vi "ziSweeper.vi"(0 "Handle In":T1 {"Handle" format="0x%08x"; "Conn" format="0x%08x"}, 1 "Output Channel (6)":u16=6 max=7, 2 "Signal Output (0)":u16 max=1, 3 "Signal Input UNUSED(0)":u16 max=1, 5 "Sweep Sequence":dbl[][](array[numeric]) format="%#_6p", 7 "Oscillator (0)":u16, 9 "Averaging":u16(ring)=1 caption="Averaging (1)" items=["1"=1, "2"=2, "4"=4, "16"=16, "32"=32, "64"=64, "128"=128], 11 "Error In":errorcluster, 12 "Input Demods (0)":u16[](array[numeric])=[0], 13 "Harmonic (1=fundamental)":i32=1 min=1 max=66000, 14 "Order (4)":i32(ring)=4 items=["6, 1st"=1, "12, 2nd"=2, "18, 3rd"=3, "24, 4th"=4, "30, 5th"=5, "36, 6th"=6, "42, 7th"=7, "48, 8th"=8]) -> (4 "Handle Out":T1 {"Handle" format="0x%08x"; "Conn" format="0x%08x"}, 6 "Output (F,X1,Y1,X2,Y2,...,Vo)":dbl[][](array[numeric]) format="%#_4p", 15 "Error Out":errorcluster)   [LabVIEW 2009, in "Zurich Instruments LabOne.lvlib"]
doc: "Perform a frequency sweep with the speciefied paramters. Use <B>ziSweepGenerator.vi</B> to generate the <B>Sweep Sequence</B>.\n\n<B>Output Channel</B> selects the channel in the output mixer that is used to generate the signal. This also determines the respective demodulator for generation of a sinusoidal.\n\nNote: <B>Signal Input</B> is only supported with the HF2LI when the Multifrequency option is installed."
uses:
  <instrlib>/Zurich Instruments LabOne/Zurich Instruments LabOne.lvlib
  <instrlib>/Zurich Instruments LabOne/Public/ziTypeHandle.ctl
  <instrlib>/Zurich Instruments LabOne/Public/Utility/ziTicksToS_single.vi
panel:
  out "Graph":cluster{dbl[], dbl[]}[](graph)
  in  "Abort":bool
  out "Remaining settle (s)":dbl caption="time to next value"
  out "Frequency":dbl caption="Frequency (Hz)" format="%_7p"
  out "Point":i32 caption="Point (#)"
  out "Progress":dbl(slide) scale=0.0..1.0
  out "Bandwidth_indic":dbl=100.0 caption="Bandwidth (Hz)" format="%_3p"
  # "Status"
  # "Progress (%)"
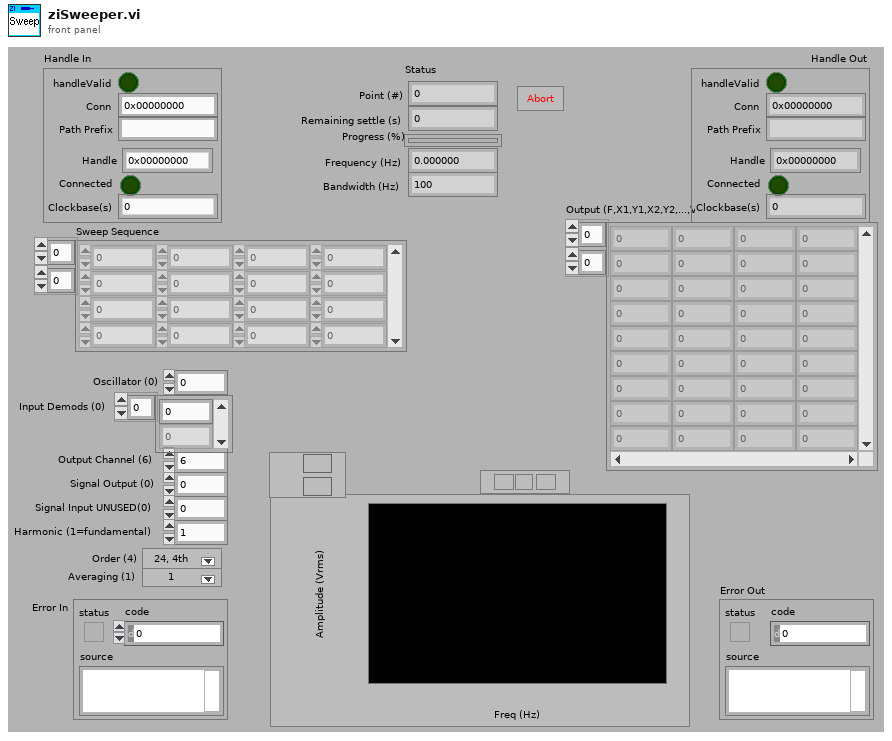
[diagram p1: front panel]
types:
  T1 = typedef "Zurich Instruments LabOne.lvlib/ziTypeHandle.ctl" = cluster{"handleValid":bool, "Conn":u64, "Path Prefix":string, "Handle":u64, "Connected":bool, "Clockbase(s)":dbl}
  T2 = cluster{"Timestamps (ticks)":u64, "X (Vrms)":dbl, "Y (Vrms)":dbl, "Osc Phase (deg)":dbl, "Freq (Hz)":dbl, "DIO":u32, "AuxIn0 (V)":dbl, "AuxIn1 (V)":dbl}
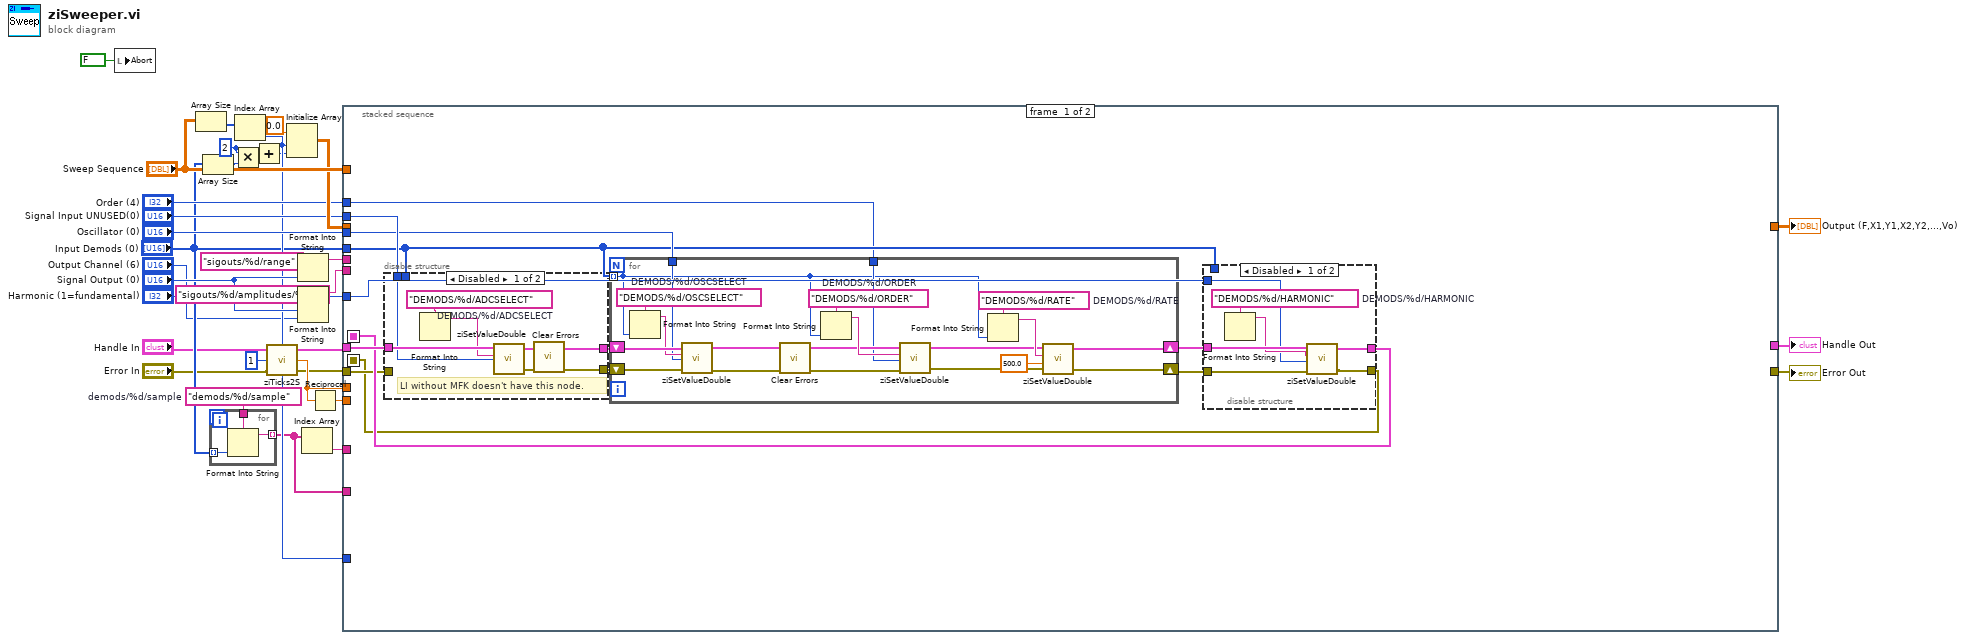
[diagram p0: block diagram]
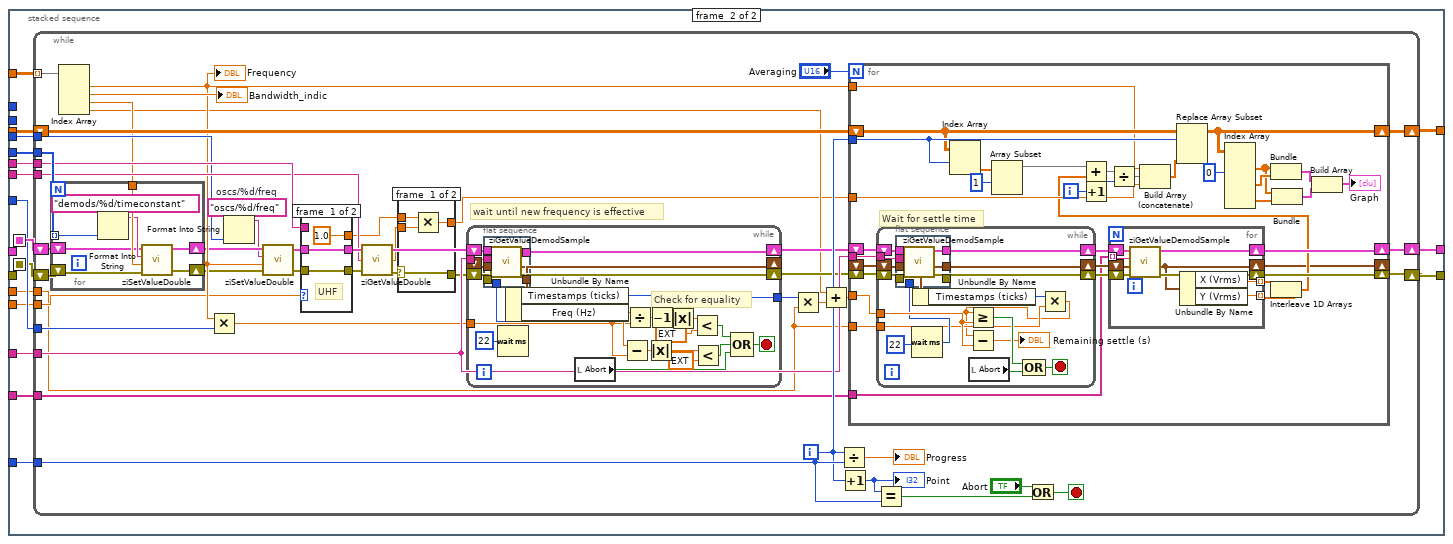
[diagram p4: hidden frame]
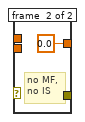
[diagram p5: hidden frame]
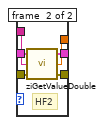
[diagram p6: hidden frame]
diagram:
  w16 = "demods/%d/sample"  # demods/%d/sample
  w9 = 2 ("dimension size")
  n1 = local write "Abort"(FALSE ("Abort")) -> ()
  n2 = Array Size(array="Sweep Sequence") -> (size(s)=w33:i32[])
  n3 = Array Size(array="Input Demods (0)") -> (size(s)=w11:i32)
  n4 = for {
    tunnel: w16 -> [w37]
    tunnel: "Input Demods (0)" -> [w36] mode=indexing
    tunnel: [w35] -> w14 mode=indexing
    n5 = Format Into String(format string=w37, w36) -> (resulting string=w35:string)  [unwired: 2 in, 1 out]
  }
  n6 = Multiply(x=w9, y=w11) -> (x*y=w10:i32)
  n7 = Index Array(array=w33) -> (element=w17:i32)  [unwired: 1 in]
  n8 = Add(x=w9, y=w10) -> (x+y=w13:i32)
  n9 = call-poly <instrlib>:"ziTicks2S.vi"("Error In"="Error In", "Timestamp(ticks)"=u64 1, "Handle In"="Handle In") -> ("Error Out"=w1:errorcluster, "Timestamp(s)"=w3:dbl, "Handle Out"=w5:T1)
  n10 = Initialize Array(0.0 ("dimension size"), w17, w13) -> (w31:dbl[][])
  n11 = Format Into String(format string="sigouts/%d/range", "Signal Output (0)") -> (resulting string=w29:string)  [unwired: 2 in, 1 out]
  n12 = Format Into String(format string="sigouts/%d/amplitudes/%d", "Signal Output (0)", "Output Channel (6)") -> (resulting string=w20:string)  [unwired: 2 in, 1 out]
  n13 = Index Array(array=w14) -> (element=w15:string)  [unwired: 1 in]
  n14 = Reciprocal(x=w3) -> (1/x=w7:dbl)
  n15 = stacked-sequence {
    seq-local: [w42 _] -> [_ w100]
    seq-local: [w39 _] -> [_ w90]
    tunnel: w31 -> [_ w104]
    tunnel: w5 -> [w50 _]
    tunnel: [_ w103] -> w25
    tunnel: [_ w102] -> w24
    tunnel: "Sweep Sequence" -> [_ w101]
    tunnel: "Input Demods (0)" -> [w46 w99]
    tunnel: w17 -> [_ w98]
    tunnel: w15 -> [_ w97]
    tunnel: w29 -> [_ w96]
    tunnel: w20 -> [_ w95]
    tunnel: [_ w94] -> w26
    tunnel: "Signal Input UNUSED(0)" -> [w48 _]
    tunnel: "Oscillator (0)" -> [w47 w92]
    tunnel: w1 -> [w40 _]
    tunnel: "Harmonic (1=fundamental)" -> [w38 w93]
    tunnel: "Order (4)" -> [w41 _]
    tunnel: w14 -> [_ w91]
    tunnel: w7 -> [_ w89]
    tunnel: w3 -> [_ w88]
    frame #0 {
      n16 = disable-structure shown="Disabled" {
        disable-tunnel: w50 -> [w56 w59]
        disable-tunnel: w48 -> [w54 _]
        disable-tunnel: w46 -> [_ _]
        disable-tunnel: [w52 w59] -> w44
        disable-tunnel: [w51 w58] -> w43
        disable-tunnel: w40 -> [_ w58]
        frame #0 {
          w57 = "DEMODS/%d/ADCSELECT"  # DEMODS/%d/ADCSELECT
          # "LI without MFK doesn't have this node."
          n17 = Format Into String(format string=w57) -> (resulting string=w55:string)  [unwired: 3 in, 1 out]
          n18 = call <instrlib>:"ziSetValueDouble.vi"("Value"=w54, "Path"=w55, "Handle In"=w56) -> ("Error Out"=w53:errorcluster, "Handle Out"=w52:T1)  [unwired: 2 in]
          n19 = call <vilib>:"Clear Errors.vi"("error in (no error)"=w53) -> ("error out"=w51:errorcluster)  [unwired: 6 in]
        }
        frame #1 {
        }
      }
      n20 = for {
        tunnel: w47 -> [w83]
        tunnel: w46 -> [w72] mode=indexing
        shift-right: [w71] -> w49
        shift-left: w44 -> [w86]
        shift-right: [w70] -> w45
        shift-left: w43 -> [w84]
        tunnel: w41 -> [w78]
        w75 = "DEMODS/%d/RATE"  # DEMODS/%d/RATE
        w82 = "DEMODS/%d/ORDER"  # DEMODS/%d/ORDER
        w87 = "DEMODS/%d/OSCSELECT"  # DEMODS/%d/OSCSELECT
        n21 = Format Into String(format string=w87, w72) -> (resulting string=w85:string)  [unwired: 2 in, 1 out]
        n22 = call <instrlib>:"ziSetValueDouble.vi"("Error In"=w84, "Value"=w83, "Path"=w85, "Handle In"=w86) -> ("Error Out"=w69:errorcluster, "Handle Out"=w80:T1)  [unwired: 1 in]
        n23 = call <vilib>:"Clear Errors.vi"("error in (no error)"=w69) -> ("error out"=w79:errorcluster)  [unwired: 6 in]
        n24 = Format Into String(format string=w82, w72) -> (resulting string=w81:string)  [unwired: 2 in, 1 out]
        n25 = call <instrlib>:"ziSetValueDouble.vi"("Error In"=w79, "Value"=w78, "Path"=w81, "Handle In"=w80) -> ("Error Out"=w74:errorcluster, "Handle Out"=w73:T1)  [unwired: 1 in]
        n26 = Format Into String(format string=w75, w72) -> (resulting string=w76:string)  [unwired: 2 in, 1 out]
        n27 = call <instrlib>:"ziSetValueDouble.vi"("Error In"=w74, "Value"=500.0 ("double precision float"), "Path"=w76, "Handle In"=w73) -> ("Error Out"=w70:errorcluster, "Handle Out"=w71:T1)  [unwired: 1 in]
      }
      n28 = disable-structure shown="Disabled" {
        disable-tunnel: w49 -> [w65 w68]
        disable-tunnel: w38 -> [w63 _]
        disable-tunnel: [w62 w68] -> w42
        disable-tunnel: [w61 w67] -> w39
        disable-tunnel: w46 -> [_ _]
        disable-tunnel: w45 -> [w60 w67]
        frame #0 {
          w66 = "DEMODS/%d/HARMONIC"  # DEMODS/%d/HARMONIC
          n29 = Format Into String(format string=w66) -> (resulting string=w64:string)  [unwired: 3 in, 1 out]
          n30 = call <instrlib>:"ziSetValueDouble.vi"("Error In"=w60, "Value"=w63, "Path"=w64, "Handle In"=w65) -> ("Error Out"=w61:errorcluster, "Handle Out"=w62:T1)  [unwired: 1 in]
        }
        frame #1 {
        }
      }
    }
    frame #1 {
      n31 = while {
        shift-right: [w152] -> w103
        shift-left: w100 -> [w115]
        shift-right: [w146] -> w102
        shift-left: w90 -> [w116]
        tunnel: w99 -> [w151]
        shift-right: [w148] -> w94
        shift-left: w104 -> [w134]
        tunnel: w101 -> [w147] mode=indexing
        tunnel: w98 -> [w137]
        tunnel: w97 -> [w130]
        tunnel: w96 -> [w145]
        tunnel: w95 -> [w144]
        tunnel: w93 -> [w143]
        tunnel: w92 -> [w142]
        tunnel: w91 -> [w114]
        tunnel: w89 -> [w106]
        tunnel: w88 -> [w105]
        i -> [w132]
        stop <- w138 stop-if-true
        w127 = "oscs/%d/freq"  # oscs/%d/freq
        # "wait until new frequency is effective"
        n32 = Index Array(array=w147) -> (element #1=w133:dbl, element #2=→"Bandwidth_indic":dbl, element #3=w131:dbl, element #4=w120:dbl)  [unwired: 4 in]
        "Frequency" <- w133
        n33 = for {
          tunnel: w151 -> [w174] mode=indexing
          tunnel: w131 -> [w173]
          shift-right: [w170] -> w125
          shift-left: w115 -> [w167]
          shift-right: [w169] -> w124
          shift-left: w116 -> [w168]
          n34 = Format Into String(format string="demods/%d/timeconstant", w174) -> (resulting string=w171:string)  [unwired: 2 in, 1 out]
          n35 = call <instrlib>:"ziSetValueDouble.vi"("Error In"=w168, "Value"=w173, "Path"=w171, "Handle In"=w167) -> ("Error Out"=w169:errorcluster, "Handle Out"=w170:T1)  [unwired: 1 in]
        }
        n36 = Multiply(x=w133, y=w143) -> (x*y=w126:dbl)
        n37 = Format Into String(format string=w127, w142) -> (resulting string=w123:string)  [unwired: 2 in, 1 out]
        n38 = call <instrlib>:"ziSetValueDouble.vi"("Error In"=w124, "Value"=w133, "Path"=w123, "Handle In"=w125) -> ("Error Out"=w117:errorcluster, "Handle Out"=w118:T1)  [unwired: 1 in]
        n39 = case shown="Default" w106 {
          tunnel: [w159 w166] -> w150
          tunnel: [w160 w165] -> w149
          tunnel: [1.0 ("Value") w164] -> w109
          tunnel: w145 -> [_ w163]
          tunnel: w118 -> [w159 w162]
          tunnel: w117 -> [w160 w161]
          frame #0 {
            # "UHF"
          }
          frame #1 {
            # "HF2"
            n40 = call <instrlib>:"ziGetValueDouble.vi"("error in"=w161, "Path"=w163, "Handle in"=w162) -> ("error out"=w165:errorcluster, "Value"=w164:dbl, "Handle out"=w166:T1)
          }
        }
        n41 = call <instrlib>:"ziGetValueDouble.vi"("error in"=w149, "Path"=w144, "Handle in"=w150) -> ("error out"=w111:errorcluster, "Value"=w108:dbl, "Handle out"=w119:T1)
        n42 = case shown="No Error" w111 {
          selector: w111 -> [w153 _]
          tunnel: w108 -> [w156 _]
          tunnel: w109 -> [w155 _]
          tunnel: [w154 0.0] -> w107
          tunnel: [w153 _] -> w110
          frame #0 {
            n43 = Multiply(x=w155, y=w156) -> (x*y=w154:dbl)
          }
          frame #1 {
            # "no MF,\nno IS"
          }
        }
        n44 = while {
          tunnel: w126 -> [w249]
          tunnel: [w266] -> w112
          shift-right: [w261] -> w128
          shift-left: w119 -> [w264]
          shift-right: [w260] -> w129
          shift-left: w110 -> [w263]
          tunnel: w130 -> [w259]
          shift-right: [w253] -> _
          shift-left: _ -> [w252]
          stop <- w265 stop-if-true
          # "Check for equality"
          n45 = flat-sequence {
            tunnel: w264 -> [w273]
            tunnel: w263 -> [w272]
            tunnel: [w271] -> w261
            tunnel: [w270] -> w260
            tunnel: w259 -> [w269]
            tunnel: [w268] -> w253
            tunnel: w252 -> [w267]
            tunnel: w244 -> [_]
            frame #0 {
              n46 = call <instrlib>:"ziGetValueDemodSample.vi"("error in"=w272, "Demod Sample In"=w267, "Path"=w269, "Handle In"=w273) -> ("error out"=w270:errorcluster, "Demod Sample Out"=w268:T2, "Handle Out"=w271:T1)  [unwired: 1 in]
            }
          }
          n47 = Wait (ms)(milliseconds to wait=22 ("timeout in ms (-1)")) -> (millisecond timer value=w244:u32)
          n48 = Unbundle By Name(w253) -> ("Timestamps (ticks)"=w266:u64, "Freq (Hz)"=w250:dbl)
          n49 = local read "Abort"() -> (w258:bool)
          n50 = Subtract(x=w250, y=w249) -> (x-y=w248:dbl)
          n51 = Divide(x=w250, y=w249) -> (x/y=w254:dbl)
          n52 = Absolute Value(x=w248) -> (abs(x)=w246:dbl)
          n53 = Decrement(x=w254) -> (x-1=w255:dbl)
          n54 = Absolute Value(x=w255) -> (abs(x)=w256:dbl)
          n55 = Less?(x=w256, y=ext 1e-7) -> (x < y?=w251:bool)
          n56 = Less?(x=w246, y=ext 0.00001) -> (x < y?=w245:bool)
          n57 = Compound Arithmetic op=OR(w251, w245, w258) -> (w265:bool)
        }
        n58 = Multiply(x=w112, y=w105) -> (x*y=w113:dbl)
        n59 = Add(x=w120, y=w113) -> (x+y=w122:dbl)
        n60 = Divide(x=w132, y=w137) -> (x/y=→"Progress":dbl)
        n61 = Increment(x=w132) -> (x+1=w135:i32)
        "Point" <- w135
        n62 = for {
          N: "Averaging" -> [_]
          shift-right: [w183] -> w152
          shift-left: w128 -> [w210]
          shift-right: [w182] -> w146
          shift-left: w129 -> [w209]
          tunnel: w122 -> [w208]
          tunnel: w107 -> [w187]
          tunnel: w133 -> [w189]
          tunnel: w132 -> [w203]
          shift-right: [w197] -> w148
          shift-left: w134 -> [w202]
          tunnel: w130 -> [w198]
          tunnel: w114 -> [w181]
          shift-right: [w177] -> _
          shift-left: _ -> [w176]
          tunnel: w105 -> [w175]
          i -> [w206]
          # "Wait for settle time"
          n63 = while {
            tunnel: w208 -> [w236]
            shift-right: [w233] -> w185
            shift-left: w209 -> [w234]
            shift-right: [w229] -> w186
            shift-left: w210 -> [w235]
            shift-right: [w227] -> w184
            shift-left: w176 -> [w228]
            tunnel: w198 -> [w225]
            tunnel: w175 -> [w221]
            stop <- w231 stop-if-true
            n64 = flat-sequence {
              tunnel: w235 -> [w243]
              tunnel: w234 -> [w242]
              tunnel: [w241] -> w233
              tunnel: [w240] -> w229
              tunnel: w228 -> [w239]
              tunnel: [w238] -> w227
              tunnel: w225 -> [w237]
              tunnel: w223 -> [_]
              frame #0 {
                n65 = call <instrlib>:"ziGetValueDemodSample.vi"("error in"=w242, "Demod Sample In"=w239, "Path"=w237, "Handle In"=w243) -> ("error out"=w241:errorcluster, "Demod Sample Out"=w238:T2, "Handle Out"=w240:T1)  [unwired: 1 in]
              }
            }
            n66 = Wait (ms)(milliseconds to wait=22 ("timeout in ms (-1)")) -> (millisecond timer value=w223:u32)
            n67 = Unbundle By Name(w227) -> ("Timestamps (ticks)"=w222:u64)
            n68 = local read "Abort"() -> (w226:bool)
            n69 = Multiply(x=w222, y=w221) -> (x*y=w220:dbl)
            n70 = Greater Or Equal?(x=w220, y=w236) -> (x >= y?=w232:bool)
            n71 = Subtract(x=w220, y=w236) -> (x-y=→"Remaining settle (s)":dbl)
            n72 = Compound Arithmetic op=OR(w232, w226) -> (w231:bool)
          }
          n73 = Index Array(array=w202, index (row)=w203) -> (element=w201:dbl[])  [unwired: 1 in]
          n74 = Array Subset(array=w201, index=1) -> (w199:dbl[])  [unwired: 1 in]
          n75 = Increment(x=w206) -> (x+1=w205:i32)
          n76 = for {
            shift-right: [w216] -> w182
            shift-left: w185 -> [w217]
            shift-right: [w215] -> w183
            shift-left: w186 -> [w218]
            tunnel: [w219] -> w180 mode=indexing
            tunnel: [w212] -> w179 mode=indexing
            shift-right: [w213] -> w177
            shift-left: w184 -> [w214]
            tunnel: w181 -> [w211] mode=indexing
            n77 = call <instrlib>:"ziGetValueDemodSample.vi"("error in"=w217, "Demod Sample In"=w214, "Path"=w211, "Handle In"=w218) -> ("error out"=w216:errorcluster, "Demod Sample Out"=w213:T2, "Handle Out"=w215:T1)  [unwired: 1 in]
            n78 = Unbundle By Name(w213) -> ("X (Vrms)"=w219:dbl, "Y (Vrms)"=w212:dbl)
          }
          n79 = Interleave 1D Arrays(w180, w179) -> (w178:dbl[])
          n80 = Add(x=w199, y=w178) -> (x+y=w207:dbl[])
          n81 = Divide(x=w207, y=w205) -> (x/y=w188:dbl[])
          n82 = Build Array (concatenate)(w189, w188, w187) -> (w204:dbl[])
          n83 = Replace Array Subset(array=w202, new element=w204, index (row)=w203) -> (w197:dbl[][])  [unwired: 1 in]
          n84 = Index Array(array=w197, index (col) #1=0 ("index (row)")) -> (element #1=w192:dbl[], element #2=w196:dbl[], element #3=w194:dbl[])  [unwired: 5 in]
          n85 = Bundle(w192, w196) -> (w195:cluster{dbl[], dbl[]})  [unwired: 1 out]
          n86 = Bundle(w192, w194) -> (w193:cluster{dbl[], dbl[]})  [unwired: 1 out]
          n87 = Build Array(w195, w193) -> (→"Graph":cluster{dbl[], dbl[]}[])
        }
        n88 = Equal?(x=w135, y=w137) -> (x = y?=w136:bool)
        n89 = Or(x="Abort", y=w136) -> (x .or. y?=w138:bool)
      }
    }
  }
  "Output (F,X1,Y1,X2,Y2,...,Vo)" <- w26
  "Handle Out" <- w25
  "Error Out" <- w24
